vi "correction.vi"(4 "electrodes/ cell":i32=5, 6 "cell length (m)":dbl=0.02 format="%#_6p", 7 "phase / 2 pi":dbl, 9 "velocity":dbl[](array[numeric]), 10 "position":dbl[](array[numeric]), 11 "time":dbl[](array[numeric])) -> (2 "frequency":dbl[](array[numeric]), 3 "waveform":dbl[](array[numeric]))   [LabVIEW 2017, in "wf.lvlib" / "wf_tools.lvlib"]
uses:
  wf_tools.lvlib
panel:
  out "frequency x":cluster{"position":dbl[], dbl[]}(graph)
  out "frequency t":cluster{"time":dbl[], dbl[]}(graph)
  out "signal x":cluster{"position":dbl[], dbl[]}(graph)
  out "signal t":cluster{"time":dbl[], dbl[]}(graph)
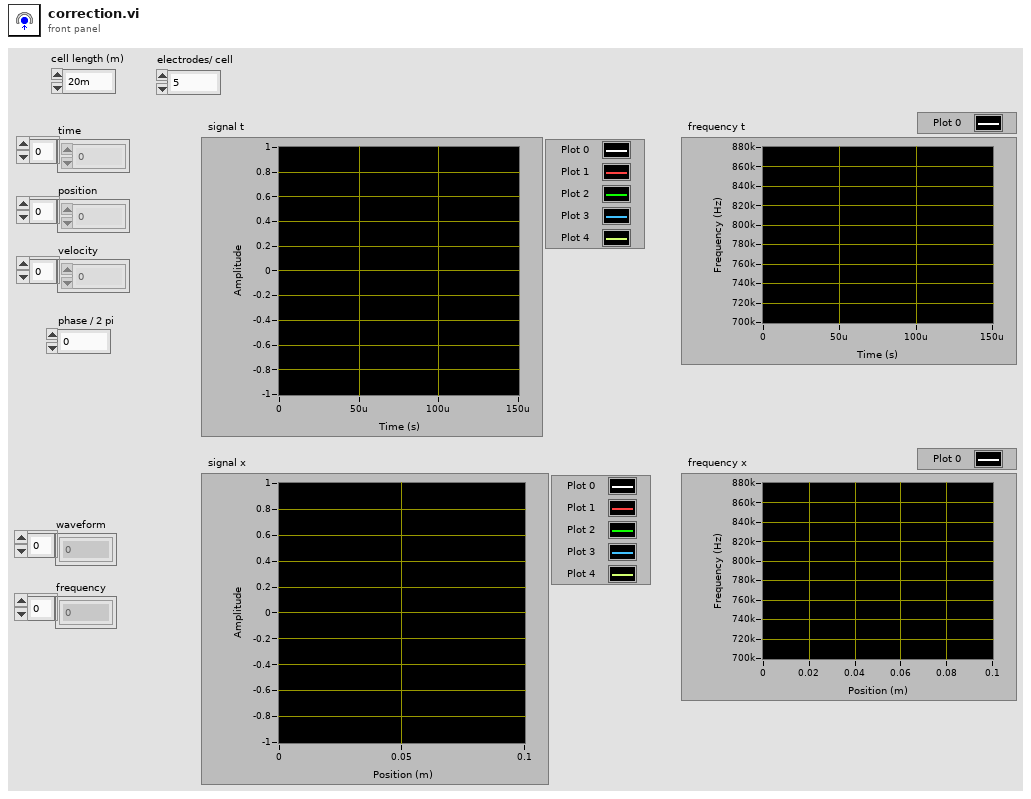
[diagram p1: front panel]
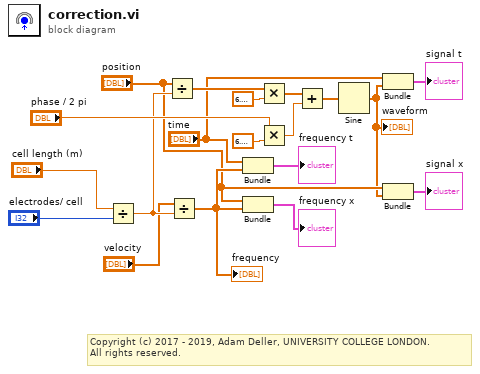
[diagram p0: block diagram]
diagram:
  # "Copyright (c) 2017 - 2019, Adam Deller, UNIVERSITY COLLEGE LONDON.\nAll rights reserved."
  n1 = Divide(x="cell length (m)", y="electrodes/ cell") -> (x/y=w8:dbl)
  n2 = Divide(x="position", y=w8) -> (x/y=w14:dbl[])
  n3 = Divide(x="velocity", y=w8) -> (x/y=w5:dbl[])
  "frequency" <- w5
  n4 = Bundle("time"="time", w5) -> (→"frequency t":cluster{"time":dbl[], dbl[]})  [unwired: 1 in]
  n5 = Bundle("position"="position", w5) -> (→"frequency x":cluster{"position":dbl[], dbl[]})  [unwired: 1 in]
  n6 = Multiply(x=w14, y=6.283185307179586) -> (x*y=w12:dbl[])
  n7 = Multiply(x="phase / 2 pi", y=6.283185307179586) -> (x*y=w9:dbl)
  n8 = Add(x=w12, y=w9) -> (x+y=w15:dbl[])
  n9 = Sine(x=w15) -> (sin(x)=w1:dbl[])
  "waveform" <- w1
  n10 = Bundle("time"="time", w1) -> (→"signal t":cluster{"time":dbl[], dbl[]})  [unwired: 1 in]
  n11 = Bundle("position"="position", w1) -> (→"signal x":cluster{"position":dbl[], dbl[]})  [unwired: 1 in]
